vi "Fpga-Top-Level-Fft-Only-Not-Ready.vi"(8 "error in":errorcluster, 11 "FFT Size":u16(ring)=16 items=["16"=16, "32"=32]) -> (0 "error out":errorcluster, 3 "Results Match!":bool)   [LabVIEW 2015]
uses:
  <vilib>/Analysis/2dsp.llb/Complex FFT.vi
  <vilib>/Analysis/NI_AALPro.lvlib
panel:
  out "Comparison failed at\nindex:":i32
  out "Expected Results (truncated)":csg[](array[numeric]) format="%#_6f"
  out "Results":csg[](array[numeric])
  out "Complex Data (in)":csg[](array[numeric])
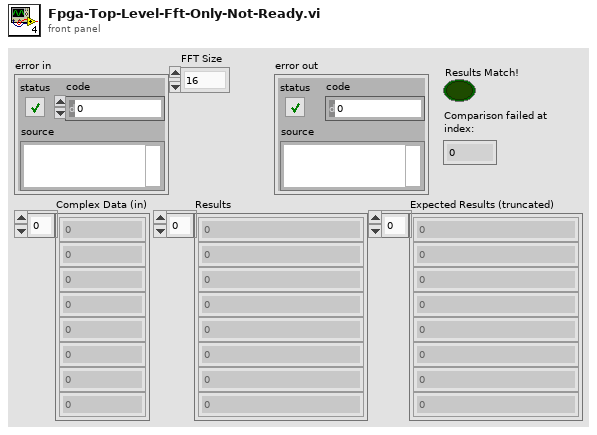
[diagram p1: front panel]
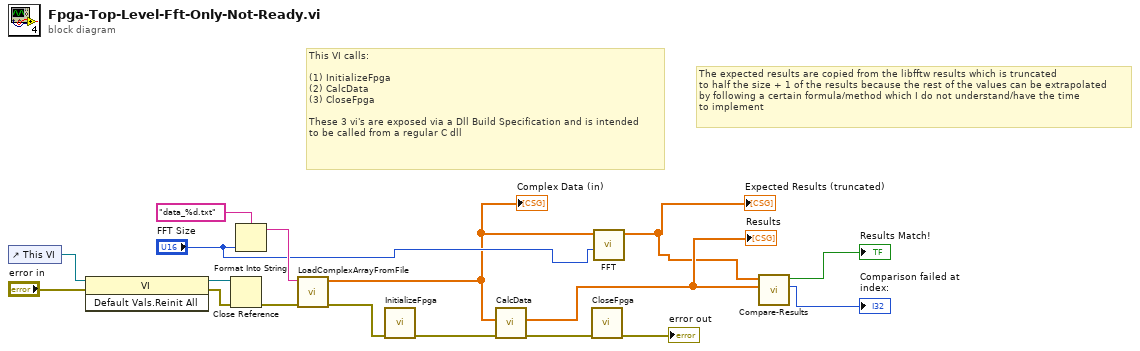
[diagram p0: block diagram]
diagram:
  # "The expected results are copied from the libfftw results which is truncated\nto half the size + 1 of the results because the rest of the values can be extrapolated\nby following a certain formula/method which I do not understand/have the time\nto implement"
  # "This VI calls:\n\n(1) InitializeFpga\n(2) CalcData\n(3) CloseFpga\n\nThese 3 vi's are exposed via a Dll Build Specification and is intended\nto be called from a regular C dll"
  n1 = control-ref of="This VI"() -> (w9:refnum<vi>)
  n2 = invoke class="VI" method="Default Vals.Reinit All"(reference=w9, error in="error in") -> (reference out=w17:refnum<vi>, error out=w16:errorcluster)  [unwired: 1 in, 1 out]
  n3 = Close Reference(reference=w17, error in (no error)=w16) -> (error out=w10:errorcluster)
  n4 = Format Into String(format string="data_%d.txt", "FFT Size") -> (resulting string=w11:string)  [unwired: 2 in, 1 out]
  n5 = call "LoadComplexArrayFromFile.vi"("error in"=w10, "SourceFileName"=w11) -> ("error out"=w13:errorcluster, "Array"=w1:csg[])  [unwired: 8 in]
  "Complex Data (in)" <- w1
  n6 = call "InitializeFpga.vi"("error in"=w13) -> ("error out"=w7:errorcluster)  [unwired: 10 in]
  n7 = call "CalcData.vi"("error in (no error)"=w7, "Complex Data (in)"=w1) -> ("error out"=w8:errorcluster, "Array out"=w4:csg[])  [unwired: 8 in]
  "Results" <- w4
  n8 = call "CloseFpga.vi"("error in"=w8) -> ("error out"=→"error out":errorcluster)  [unwired: 10 in]
  n9 = call-poly <vilib>:"FFT.vi"("FFT size"="FFT Size", "X"=w1) -> ("FFT {X}"=w3:cdb[])  [unwired: 8 in, 1 out]
  "Expected Results (truncated)" <- w3
  n10 = call "Compare-Results.vi"("FFT {X}"=w4, "Array in"=w3) -> ("Numeric"=→"Comparison failed at\nindex:":i32, "Boolean"=→"Results Match!":bool)  [unwired: 8 in]
